vi "Write SA Pin.vi"(8 "error in (no error)":errorcluster, 10 "SA Pin":string, 11 "NR_ACP in":refnum<class "NR_ACP.lvclass">) -> (0 "error out":errorcluster, 3 "NR_ACP out":refnum<class "NR_ACP.lvclass">)   [LabVIEW 2018, in "SeqAuto Evaluations.lvlib" / "NR_ACP.lvclass"]
uses:
  NR_ACP.lvclass
  NR_ACP.lvclass/NR_ACP.ctl
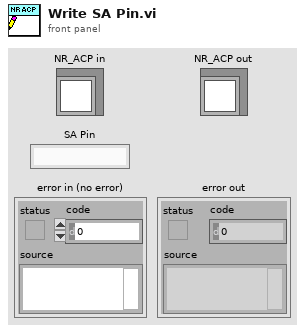
[diagram p1: front panel]
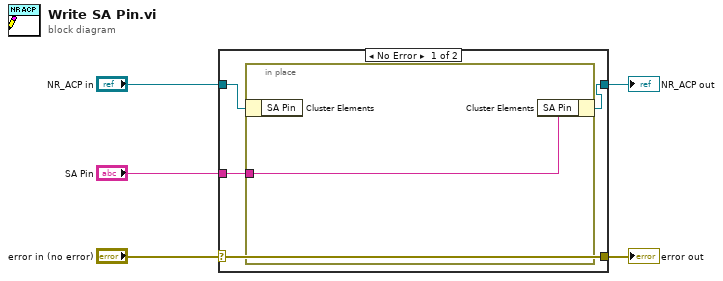
[diagram p0: block diagram]
diagram:
  n1 = case shown="No Error" "error in (no error)" {
    selector: "error in (no error)" -> [w9 w11]
    tunnel: [w9 w11] -> w4
    tunnel: [w6 w12] -> w2
    tunnel: "NR_ACP in" -> [w7 w12]
    tunnel: "SA Pin" -> [w8 _]
    frame No Error {
      n2 = in-place {
        in-place-border: w8 -> [w10]
        n3 = in-place-cluster #1(w7) -> ()  [unwired: 1 out]
        n4 = in-place-cluster #1("SA Pin"=w10) -> (w6:refnum<class "NR_ACP.lvclass">)
      }
    }
    frame Error {
    }
  }
  "error out" <- w4
  "NR_ACP out" <- w2
